vi "Add Starting Value to DB.vi"(0 "Test Number and Bin Generator In":refnum<class "Test Number and Bin Generator.lvclass">=refnum, 11 "error in (no error)":errorcluster) -> (4 "Test Number and Bin Generator Out":refnum<class "Test Number and Bin Generator.lvclass">, 15 "error out":errorcluster)   [LabVIEW 2018, in "Test Number and Bin Generator.lvlib" / "Test Number and Bin Generator.lvclass"]
uses:
  Test Number and Bin Generator.lvclass
  Test Number and Bin Generator.lvclass/Test Number and Bin Generator.ctl
  Test Group/Test Group.lvclass
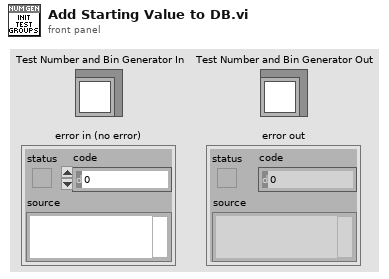
[diagram p1: front panel]
types:
  T1 = typedef "Test Number and Bin Generator.lvlib/Test Number and Bin Generator.lvclass/Test Group.ctl" = cluster{"Test Group Name":string, "Starting Number":i32, "Number of Elements":i32}
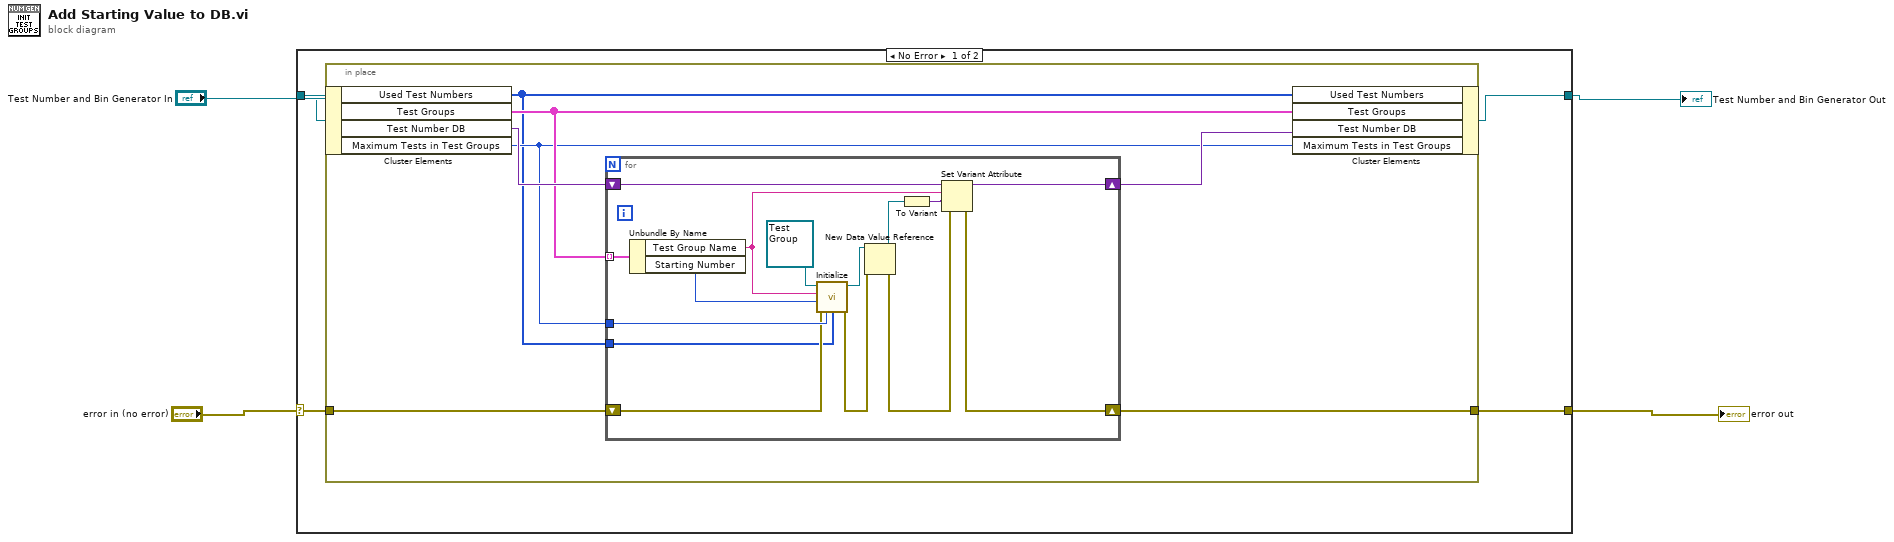
[diagram p0: block diagram]
diagram:
  n1 = case shown="No Error" "error in (no error)" {
    selector: "error in (no error)" -> [w5 w32]
    tunnel: "Test Number and Bin Generator In" -> [w8 w31]
    tunnel: [w7 w32] -> w4
    tunnel: [w6 w31] -> w1
    frame No Error {
      n2 = in-place {
        in-place-border: [w14] -> w7
        in-place-border: w5 -> [w15]
        n3 = in-place-cluster #1(w8) -> ("Used Test Numbers"=w9:i64[], "Test Groups"=w11:T1[], "Test Number DB"=w13:variant, "Maximum Tests in Test Groups"=w10:i32)
        n4 = for {
          shift-right: [w23] -> w14
          shift-left: w15 -> [w25]
          tunnel: w11 -> [w30] mode=indexing
          shift-right: [w24] -> w12
          shift-left: w13 -> [w29]
          tunnel: w10 -> [w26]
          tunnel: w9 -> [w22]
          n5 = Unbundle By Name(w30) -> ("Test Group Name"=w28:string, "Starting Number"=w27:i32)
          n6 = call "Initialize.vi"("Numbers to Exlude"=w22, "Max Number of Tests"=w26, "error in (no error)"=w25, "Starting Value"=w27, "Name"=w28, "Test Group in"=refnum<class "Test Group.lvclass"> refnum) -> ("error out"=w20:errorcluster, "Test Group out"=w21:refnum<class "Test Group.lvclass">)  [unwired: 4 in]
          n7 = New Data Value Reference(data value=w21, error in=w20) -> (data value reference=w18:refnum<data-value>, error out=w19:errorcluster)
          n8 = To Variant(anything=w18) -> (Variant=w17:variant)
          n9 = Set Variant Attribute(Variant=w29, name=w28, value=w17, error in=w19) -> (Variant out=w24:variant, error out=w23:errorcluster)  [unwired: 1 out]
        }
        n10 = in-place-cluster #1("Used Test Numbers"=w9, "Test Groups"=w11, "Test Number DB"=w12, "Maximum Tests in Test Groups"=w10) -> (w6:refnum<class "Test Number and Bin Generator.lvclass">)
      }
    }
    frame Error {
    }
  }
  "error out" <- w4
  "Test Number and Bin Generator Out" <- w1
